vi "callTCV.vi"() -> ()   [LabVIEW 2024]
uses:
  dependencies_dll_release/TCV_Lib.dll
panel:
  out "arry_cluster":T1(array[cluster])
  out "no_of_detections":i32
  in  "CPU:0/Gpu:1":i32=1
  in  "camIndex":i32
  out "class_name_success":i32
  in  "Class name path":path=path "D:/labviewTestTCVdll/TransformCV-LabVIEW/Test/model/classes.txt"
  out "Device Num":u64
  out "success_model_loading":u64
  in  "Model Path":path=path "D:/labviewTestTCVdll/TransformCV-LabVIEW/Test/model/nws_736_1280_b1_gpu.torchscript"
  in  "Image Path":path=path "D:/labviewTestTCVdll/TransformCV-LabVIEW/Test/model/test_img.jpg"
  in  "model_h":i32=736
  in  "iou":dbl=0.6
  in  "conf":dbl=0.4
  in  "frame_w":i32=1280
  in  "frame_h":i32=736
  in  "model_w":i32=1280
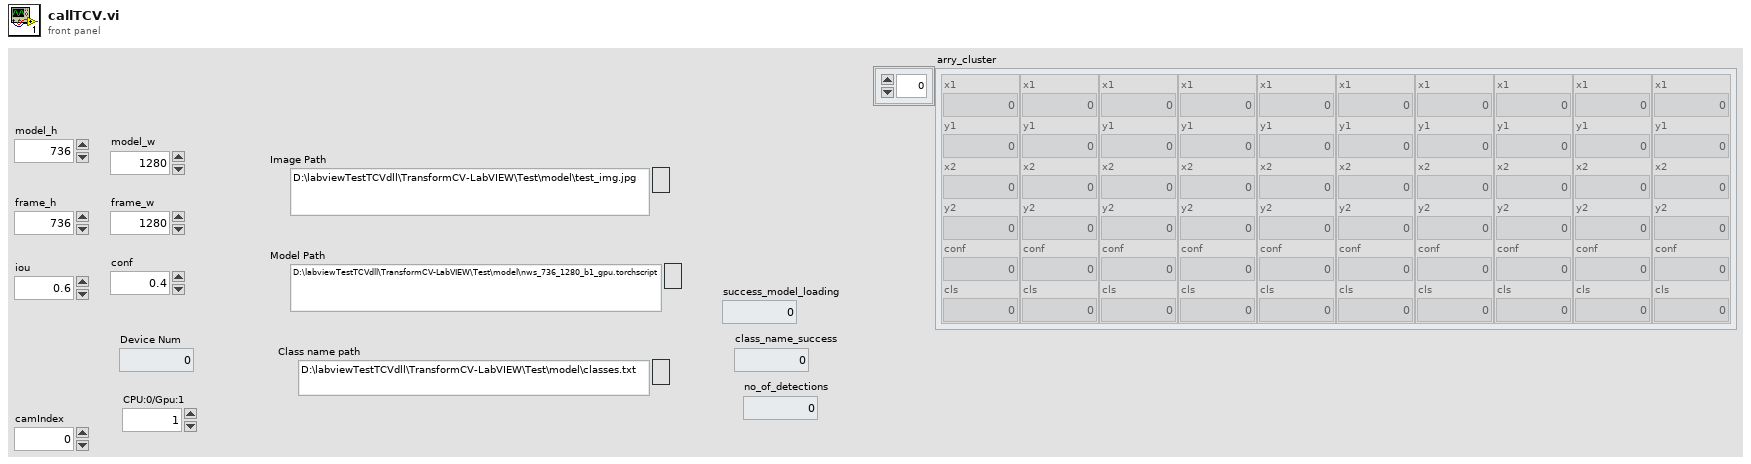
[diagram p1: front panel]
types:
  T1 = cluster{"x1":sgl, "y1":sgl, "x2":sgl, "y2":sgl, "conf":sgl, "cls":i32}[]
  T2 = cluster{"x1":sgl, "y1":sgl, "x2":sgl, "y2":sgl, "conf":sgl, "cls":i32}
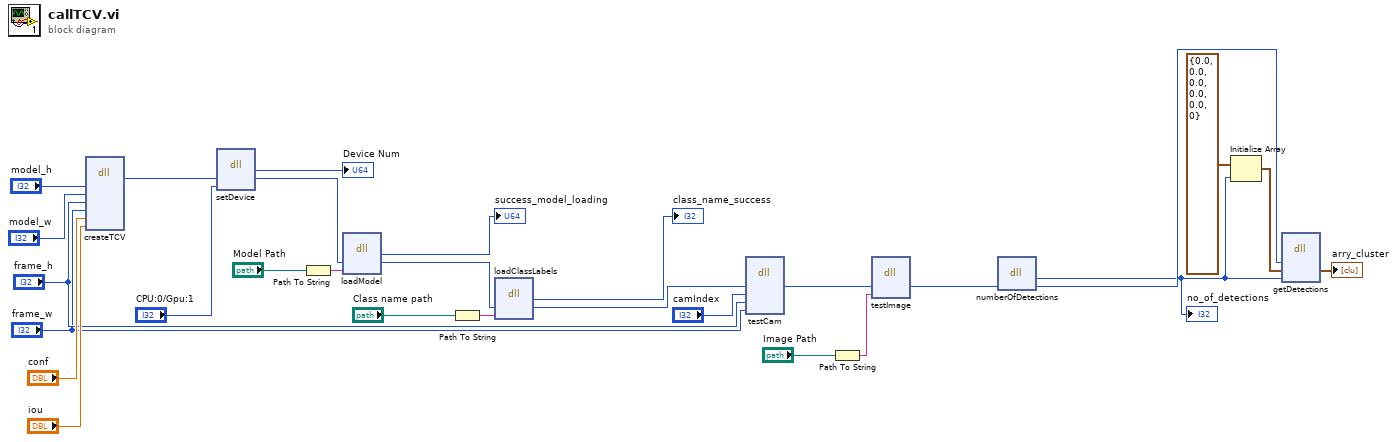
[diagram p0: block diagram]
diagram:
  n1 = dll-call lib="D:/labviewTestTCVdll/TransformCV-LabVIEW/Test/dependencies_dll_release/TCV_Lib.dll" fn="createTCV"("model_h"="model_h", "model_w"="model_w", "frame_h"="frame_h", "frame_w"="frame_w", "conf"="conf", "iou"="iou") -> ("return Obj"=w20:u64)  [unwired: 9 in, 2 out]
  n2 = dll-call lib="D:/labviewTestTCVdll/TransformCV-LabVIEW/Test/dependencies_dll_release/TCV_Lib.dll" fn="setDevice"("ref"=w20, "device"="CPU:0/Gpu:1") -> ("return type"=→"Device Num":u64, "ref"=w17:u64)  [unwired: 4 in, 2 out]
  n3 = Path To String(path="Model Path") -> (string=w21:string)
  n4 = dll-call lib="D:/labviewTestTCVdll/TransformCV-LabVIEW/Test/dependencies_dll_release/TCV_Lib.dll" fn="loadModel"("ref"=w17, "path"=w21) -> ("success"=→"success_model_loading":u64, "ref"=w14:u64)  [unwired: 4 in, 2 out]
  n5 = Path To String(path="Class name path") -> (string=w15:string)
  n6 = dll-call lib="D:/labviewTestTCVdll/TransformCV-LabVIEW/Test/dependencies_dll_release/TCV_Lib.dll" fn="loadClassLabels"("ref"=w14, "class_names"=w15) -> ("return type"=→"class_name_success":i32, "ref"=w12:u64)  [unwired: 4 in, 2 out]
  n7 = dll-call lib="D:/labviewTestTCVdll/TransformCV-LabVIEW/Test/dependencies_dll_release/TCV_Lib.dll" fn="testCam"("ref"=w12, "camIndex"="camIndex", "h"="frame_h", "w"="frame_w") -> ("ref"=w10:u64)  [unwired: 7 in, 2 out]
  n8 = Path To String(path="Image Path") -> (string=w23:string)
  n9 = dll-call lib="D:/labviewTestTCVdll/TransformCV-LabVIEW/Test/dependencies_dll_release/TCV_Lib.dll" fn="testImage"("ref"=w10, "path"=w23) -> ("ref"=w6:u64)  [unwired: 5 in, 2 out]
  n10 = dll-call lib="D:/labviewTestTCVdll/TransformCV-LabVIEW/Test/dependencies_dll_release/TCV_Lib.dll" fn="numberOfDetections"("ref"=w6) -> ("no_of_detections"=w2:i32, "ref"=w4:u64)  [unwired: 3 in, 2 out]
  "no_of_detections" <- w2
  n11 = Initialize Array(T2 {"x1"=0.0, "y1"=0.0, "x2"=0.0, "y2"=0.0, "conf"=0.0, "cls"=0}, w2) -> (w3:T1)
  n12 = dll-call lib="D:/labviewTestTCVdll/TransformCV-LabVIEW/Test/dependencies_dll_release/TCV_Lib.dll" fn="getDetections"("ref"=w4, "arry_cluster"=w3, "numberofdetection"=w2) -> ("arry_cluster"=→"arry_cluster":T1)  [unwired: 6 in, 2 out]
